vi "StateDrivebase.vi"(0 "Master State":T1(ring)) -> ()   [LabVIEW 2019]
doc: "This VI performs all of the calculations and decisions related to the swerve drive. Driver profiles are tuned from this front panel."
uses:
  <vilib>/Rock Robotics/WPI/DriverStation/WPI_DriverStationRobotMode2.ctl
  dscommands.vi
  constants.vi
  dsdata.vi
  sensors.vi
  outputs.vi
panel:
  in  "Manual Fudge Factor Auto Target (deg)":dbl=5.0
  in  "PID Tuning Heading Lock":T2={"Kp"=0.00045, "Ki"=0.0, "Kd"=0.0, "N-Diff"=3, "N-Int"=10, "Int Error Window"=90.0, "Max Ouput"=1.0, "Min Output"=-1.0, "Square Derivative"=FALSE, "N-Prop"=5} {"N-Prop" min=1; "Int Error Window" min=0.0; "N-Int" min=2; "N-Diff" min=2; "Kd" min=0.0; "Ki" min=0.0; "Kp" min=0.0}
  in  "Deceleration Hysteresis (ms)":u32=1
  out "Heading Control":bool
  in  "Heading Lock Strafe Deadband (ft/s)":dbl=3.0
  in  "Manually Disable Heading Lock":bool
  in  "PID Tuning Feeder Station":T3={"Kp"=0.0045, "Ki"=0.01, "Kd"=0.0002, "N-Diff"=10, "N-Int"=10, "Int Error Window"=30.0, "Max Ouput"=1.0, "Min Output"=-1.0} {"Int Error Window" min=0.0; "N-Int" min=2; "N-Diff" min=2; "Kd" min=0.0; "Ki" min=0.0; "Kp" min=0.0}
  out "Heading Controller Summary":T4(graph)
  in  "PID Tuning Auto Targeting":T3={"Kp"=0.006, "Ki"=0.0, "Kd"=0.0002, "N-Diff"=10, "N-Int"=10, "Int Error Window"=30.0, "Max Ouput"=0.4, "Min Output"=-0.4} {"Int Error Window" min=0.0; "N-Int" min=2; "N-Diff" min=2; "Kd" min=0.0; "Ki" min=0.0; "Kp" min=0.0}
  in  "Manual Fudge Factor Feeder Station(deg)":dbl=10.0
  in  "Plot Heading PID":bool
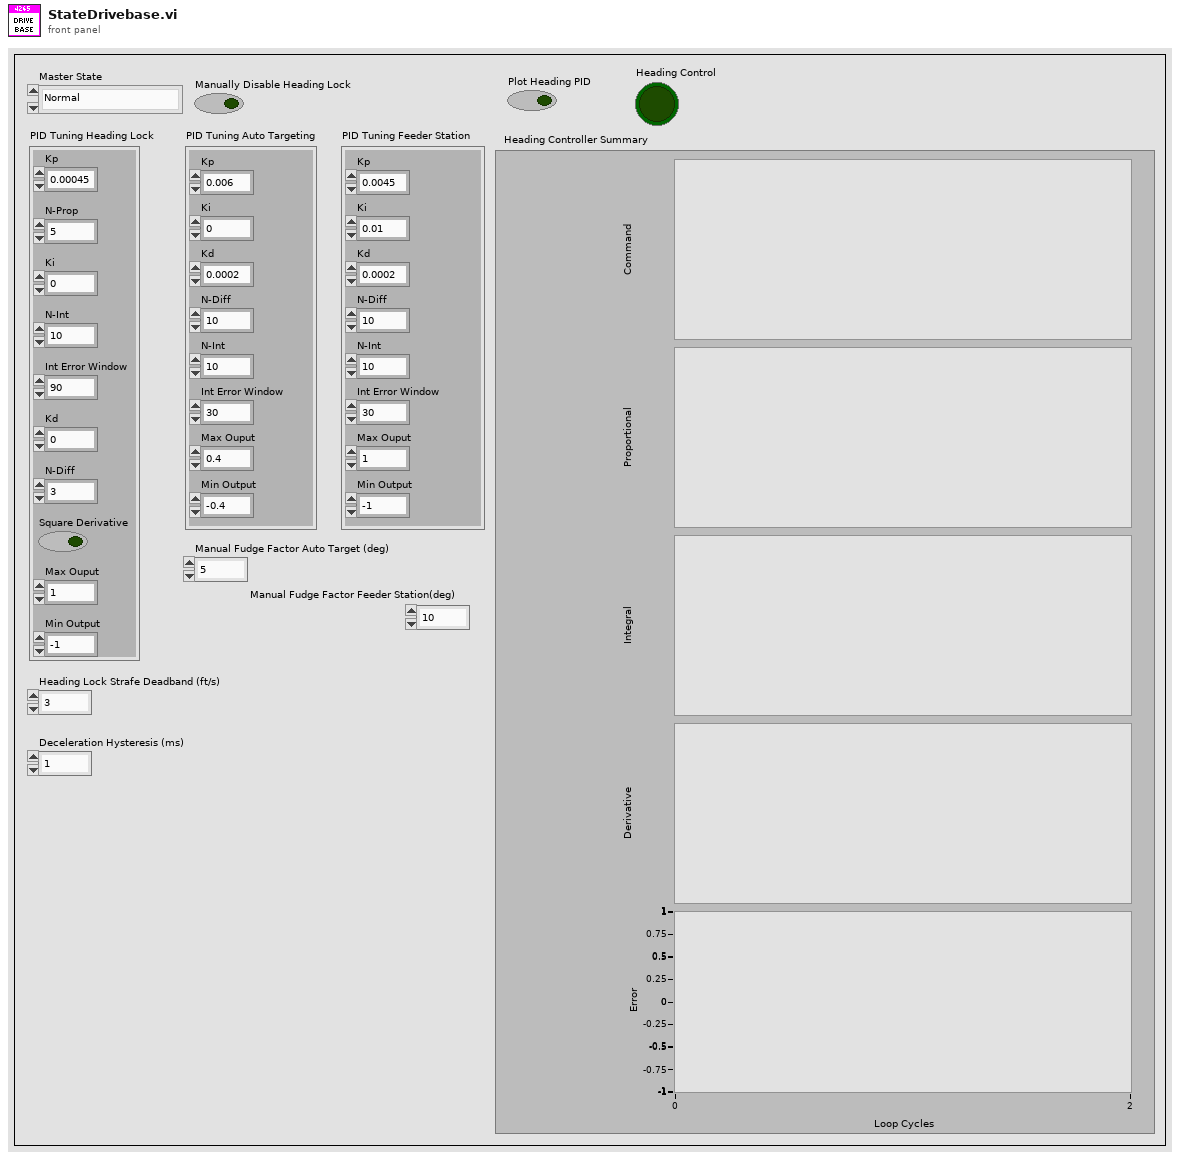
[diagram p1: front panel]
types:
  T1 = enum16{"Normal", "Control Rotation", "Control Position", "Climb"}
  T2 = cluster{"Kp":dbl, "Ki":dbl, "Kd":dbl, "N-Diff":i32, "N-Int":i32, "Int Error Window":dbl, "Max Ouput":dbl, "Min Output":dbl, "Square Derivative":bool, "N-Prop":i32}
  T3 = cluster{"Kp":dbl, "Ki":dbl, "Kd":dbl, "N-Diff":i32, "N-Int":i32, "Int Error Window":dbl, "Max Ouput":dbl, "Min Output":dbl}
  T4 = cluster{"Command":dbl, "Proportional":dbl, "Integral":dbl, "Derivative":dbl, "Goal":dbl}
  T5 = enum16{"Driver Control", "Auto Targeting", "Feeder Station"}
  T6 = typedef "WPI_DriverStationRobotMode2.ctl" = enum16{"Autonomous Disabled", "Autonomous Enabled", "Teleop Disabled", "Teleop Enabled", "Disconnected", "Finish", "Test Disabled", "Test Enabled", "Emergency Stopped"}
  T7 = cluster{"Current Setpoints[0]":dbl, "Current Setpoints[1]":dbl, "Current Setpoints[2]":dbl, "Current Setpoints[3]":dbl, "Current Setpoints[4]":dbl, "Current Setpoints[5]":dbl, "Current Setpoints[6]":dbl, "Current Setpoints[7]":dbl, "Current Setpoints[8]":dbl}
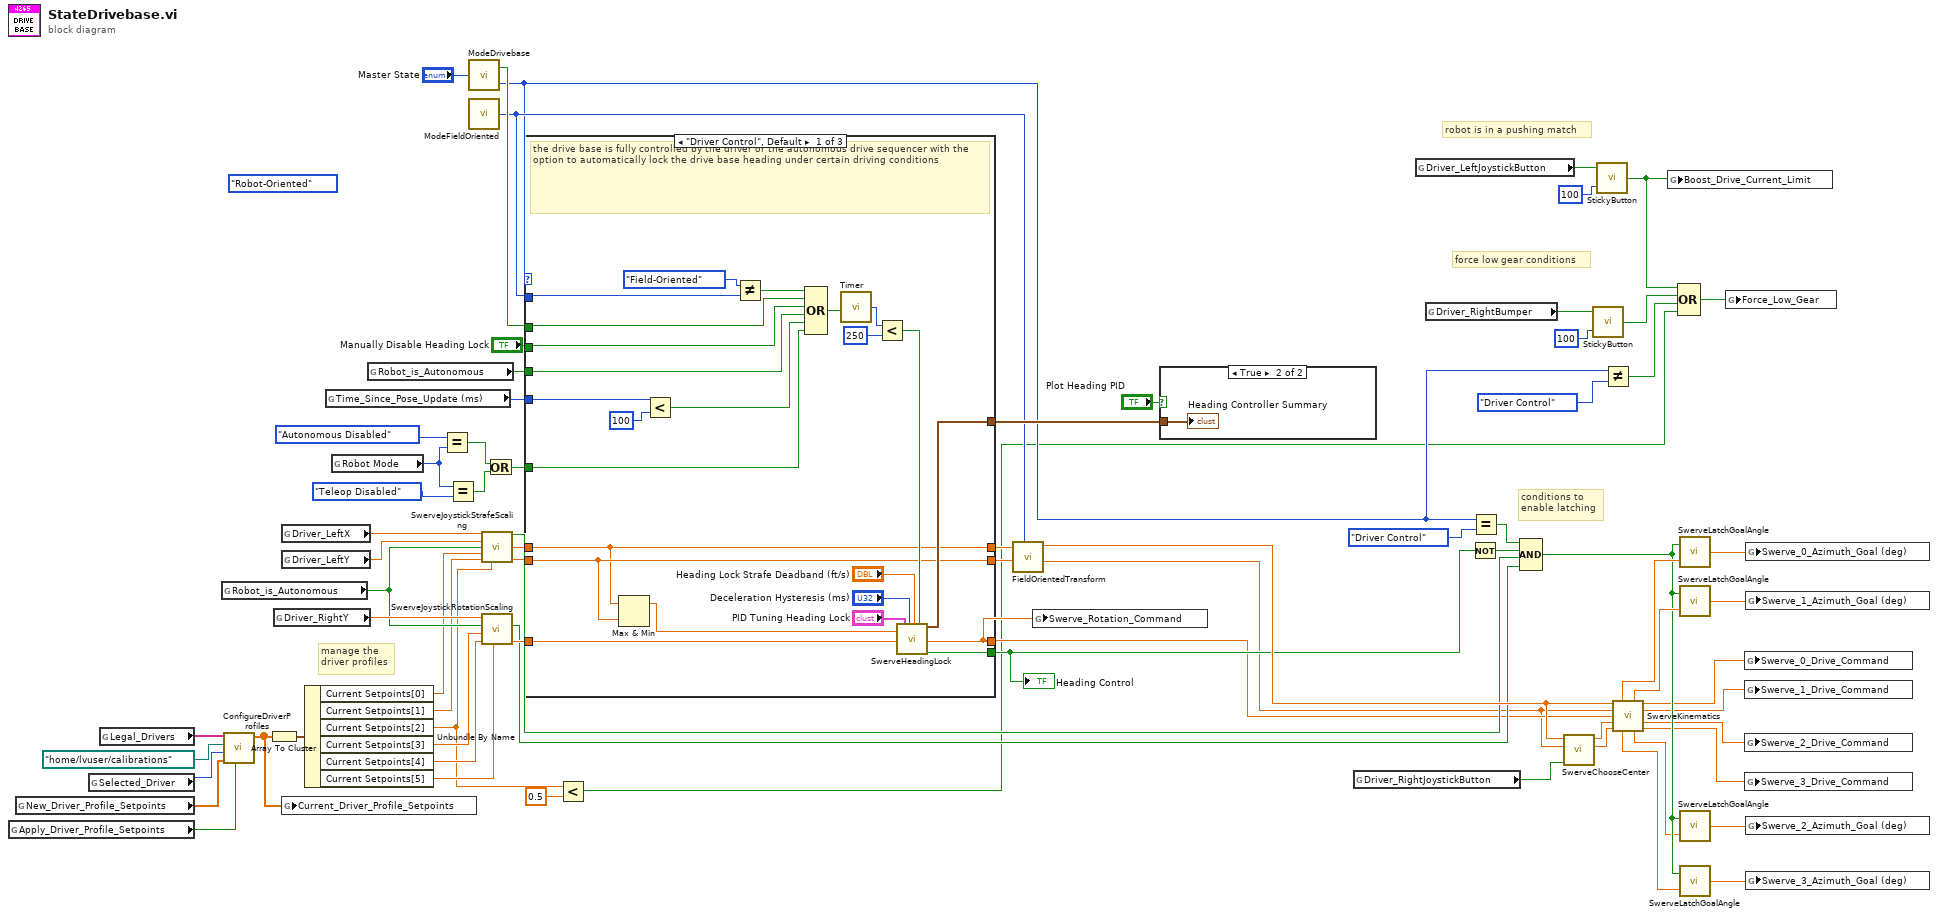
[diagram p0: block diagram]
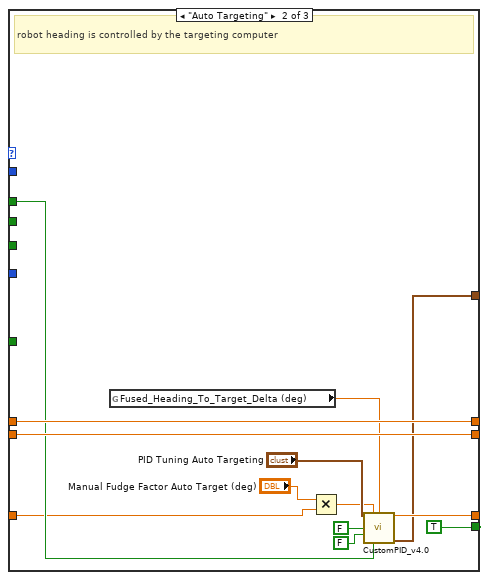
[diagram p3: hidden frame]
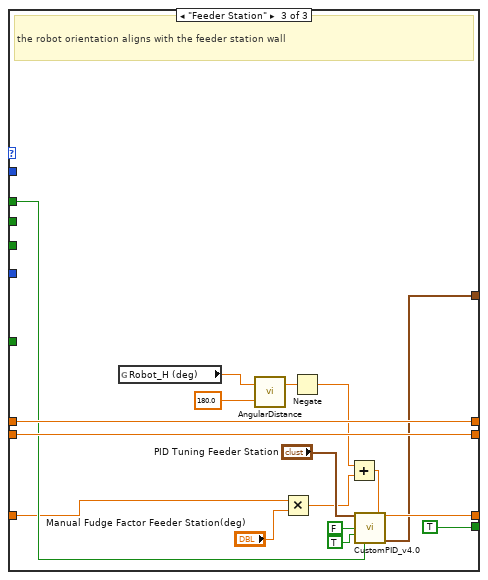
[diagram p4: hidden frame]
diagram:
  (unwired) enum16{"Robot-Oriented", "Field-Oriented"}."Robot-Oriented" ("Orientation Mode")
  # "force low gear conditions"
  # "robot is in a pushing match"
  # "conditions to\nenable latching"
  # "manage the\ndriver profiles"
  n1 = global read "dsdata.vi" "Apply_Driver_Profile_Setpoints"() -> (w7:bool)
  n2 = global read "dsdata.vi" "New_Driver_Profile_Setpoints"() -> (w9:dbl[])
  n3 = global read "dsdata.vi" "Selected_Driver"() -> (w8:i32)
  n4 = global read "constants.vi" "Legal_Drivers"() -> (w11:string[])
  n5 = global read "dsdata.vi" "Robot_is_Autonomous"() -> (w52:bool)
  n6 = call "ConfigureDriverProfiles.vi"("Apply New Setpoint"=w7, "New Setpoints"=w9, "Selected Driver"=w8, "Setpoint Save Location"=path "/home/lvuser/calibrations", "Driver Profile Names"=w11) -> ("Current Setpoints"=w6:dbl[])  [unwired: 6 in]
  n7 = Array To Cluster(array=w6) -> (cluster=w5:T7)
  n8 = global read "dscommands.vi" "Driver_RightY"() -> (w53:dbl)
  n9 = global read "dscommands.vi" "Driver_LeftX"() -> (w58:dbl)
  n10 = global read "dscommands.vi" "Driver_LeftY"() -> (w57:dbl)
  n11 = global write "outputs.vi" "Current_Driver_Profile_Setpoints"(w6) -> ()
  n12 = Unbundle By Name(w5) -> ("Current Setpoints[0]"=w40:dbl, "Current Setpoints[1]"=w39:dbl, "Current Setpoints[2]"=w3:dbl, "Current Setpoints[3]"=w24:dbl, "Current Setpoints[4]"=w23:dbl, "Current Setpoints[5]"=w22:dbl)
  n13 = global read "sensors.vi" "Time_Since_Pose_Update (ms)"() -> (w66:u32)
  n14 = global read "dsdata.vi" "Robot Mode"() -> (w29:T6)
  n15 = global read "dsdata.vi" "Robot_is_Autonomous"() -> (w65:bool)
  n16 = Equal?(x=WPI_DriverStationRobotMode2."Autonomous Disabled" ("Robot Mode"), y=w29) -> (x = y?=w27:bool)
  n17 = Equal?(x=w29, y=WPI_DriverStationRobotMode2."Teleop Disabled" ("Robot Mode")) -> (x = y?=w26:bool)
  n18 = call "ModeDrivebase.vi"("Master State"="Master State") -> ("Drive Mode Change"=w63:bool, "Drive Mode"=w14:T5)
  n19 = call "ModeFieldOriented.vi"() -> ("Orientation Mode"=w42:enum16{"Robot-Oriented", "Field-Oriented"})  [unwired: 1 in]
  n20 = call "SwerveJoystickStrafeScaling.vi"("Raw Joystick X"=w58, "Raw Joystick Y"=w57, "Auto Control"=w52, "Strafe Deadband"=w40, "Strafe Scaling"=w39, "Strafe Maximum"=w3) -> ("In Deadband"=w48:bool, "Scaled Joystick X"=w56:dbl, "Scaled Joystick Y"=w55:dbl)  [unwired: 7 in]
  n21 = call "SwerveJoystickRotationScaling.vi"("Rotation Maximum"=w22, "Rotation Scaling"=w23, "Rotation Deadband"=w24, "Auto Control"=w52, "Raw Joystick Rotation"=w53) -> ("Scaled Joystick Rotation"=w54:dbl, "In Deadband"=w49:bool)  [unwired: 4 in]
  n22 = Or(x=w27, y=w26) -> (x .or. y?=w25:bool)
  n23 = case shown="\"Driver Control\", Default" w14 {
    tunnel: [w76 w109 w125] -> w41
    tunnel: [w75 w110 w123] -> w73
    tunnel: w56 -> [w75 w110 w123]
    tunnel: w55 -> [w76 w109 w125]
    tunnel: w54 -> [w87 w99 w115]
    tunnel: [w88 w101 w122] -> w47
    tunnel: [w93 TRUE ("auto rot control") TRUE ("auto rot control")] -> w50
    tunnel: w42 -> [w94 _ _]
    tunnel: w65 -> [w91 _ _]
    tunnel: w63 -> [w85 w104 w118]
    tunnel: w66 -> [w97 _ _]
    tunnel: [w90 w100 w117] -> w64
    tunnel: "Manually Disable Heading Lock" -> [w89 _ _]
    tunnel: w25 -> [w79 _ _]
    frame "Driver Control", Default {
      # "the drive base is fully controlled by the driver or the autonomous drive sequencer with the option to automatically lock the drive base heading under certain driving conditions"
      n24 = Max & Min(x=w75, y=w76) -> (max(x,y)=w74:dbl)  [unwired: 1 out]
      n25 = Less?(x=w97, y=u32 100) -> (x < y?=w92:bool)
      n26 = Not Equal?(x=enum16{"Robot-Oriented", "Field-Oriented"}."Field-Oriented" ("Orientation Mode"), y=w94) -> (x != y?=w84:bool)
      n27 = Compound Arithmetic op=OR(w84, w85, w89, w91, w92, w79) -> (w82:bool)
      n28 = call "Timer.vi"("Reset Timer"=w82) -> ("Time (ms)"=w83:u32)
      n29 = Less?(x=w83, y=u32 250) -> (x < y?=w80:bool)
      n30 = call "SwerveHeadingLock.vi"("Max Driver Translation Joystick"=w74, "Driver Rotation Joystick"=w87, "PID Tuning Parameters"="PID Tuning Heading Lock", "Deceleration Hysteresis (ms)"="Deceleration Hysteresis (ms)", "Heading Lock Strafe Deadband (ft/s)"="Heading Lock Strafe Deadband (ft/s)", "External Disables"=w80) -> ("Controller Summary"=w90:T4, "Joystick Rotation"=w88:dbl, "Heading Lock"=w93:bool)  [unwired: 11 in]
    }
    frame "Auto Targeting" {
      # "robot heading is controlled by the targeting computer"
      n31 = global read "sensors.vi" "Fused_Heading_To_Target_Delta (deg)"() -> (w105:dbl)
      n32 = Multiply(x="Manual Fudge Factor Auto Target (deg)", y=w99) -> (x*y=w106:dbl)
      n33 = call "CustomPID_v4.0.vi"("PID Tuning Parameters"="PID Tuning Auto Targeting", "Goal"=w106, "Process Variable"=w105, "Reset on Goal Change ?"=FALSE, "Use Custom Error Calculation ?"=FALSE, "Reinit"=w104) -> ("Command"=w101:dbl, "Controller Summary"=w100:T4)  [unwired: 6 in, 2 out]
    }
    frame "Feeder Station" {
      # "the robot orientation aligns with the feeder station wall"
      n34 = global read "sensors.vi" "Robot_H (deg)"() -> (w127:dbl)
      n35 = call "AngularDistance.vi"("Goal Angle (deg) [0,360]"=180.0, "Current Angle (deg) [-Inf,+Inf]"=w127) -> ("Signed Angular Distance (deg) [-180,+180]"=w116:dbl)  [unwired: 1 out]
      n36 = Multiply(x=w115, y="Manual Fudge Factor Feeder Station(deg)") -> (x*y=w114:dbl)
      n37 = Negate(x=w116) -> (-x=w113:dbl)
      n38 = Add(x=w113, y=w114) -> (x+y=w112:dbl)
      n39 = call "CustomPID_v4.0.vi"("PID Tuning Parameters"="PID Tuning Feeder Station", "Custom Error Calculation"=w112, "Reset on Goal Change ?"=FALSE, "Use Custom Error Calculation ?"=TRUE, "Reinit"=w118) -> ("Command"=w122:dbl, "Controller Summary"=w117:T4)  [unwired: 7 in, 2 out]
    }
  }
  "Heading Control" <- w50
  n40 = Less?(x=w3, y=0.5) -> (x < y?=w1:bool)
  n41 = call "FieldOrientedTransform.vi"("Orientation Mode"=w42, "Joystick Y"=w41, "Joystick X"=w73) -> ("Joystick Y'"=w43:dbl, "Joystick X'"=w51:dbl)  [unwired: 7 in]
  n42 = global write "outputs.vi" "Swerve_Rotation_Command"(w47) -> ()
  n43 = case shown="True" "Plot Heading PID" {
    tunnel: w64 -> [_ w128]
    frame False {
    }
    frame True {
      "Heading Controller Summary" <- w128
    }
  }
  n44 = global read "dscommands.vi" "Driver_RightJoystickButton"() -> (w62:bool)
  n45 = global read "dscommands.vi" "Driver_LeftJoystickButton"() -> (w60:bool)
  n46 = global read "dscommands.vi" "Driver_RightBumper"() -> (w21:bool)
  n47 = Not(x=w50) -> (.not. x?=w46:bool)
  n48 = Equal?(x=w14, y=T5."Driver Control" ("x")) -> (x = y?=w45:bool)
  n49 = Compound Arithmetic op=AND(w45, w46, w48, w49) -> (w69:bool)
  n50 = call "SwerveChooseCenter.vi"("Defensive Driving Trigger"=w62, "Joystick Y"=w43, "Joystick X"=w51) -> ("Cy (in)"=w12:dbl, "Cx (in)"=w13:dbl)  [unwired: 5 in]
  n51 = call "StickyButton.vi"("Time threshold (ms)"=u32 100 ("y"), "Button Input"=w21) -> ("Sticky Button"=w18:bool)
  n52 = call "StickyButton.vi"("Time threshold (ms)"=u32 100 ("y"), "Button Input"=w60) -> ("Sticky Button"=w19:bool)
  n53 = Not Equal?(x=w14, y=T5."Driver Control") -> (x != y?=w15:bool)
  n54 = call "SwerveKinematics.vi"("Joystick X"=w51, "Joystick Y"=w43, "Joystick Rotation"=w47, "Cx (in)"=w13, "Cy (in)"=w12) -> ("Module 0 Angle (deg)"=w72:dbl, "Module 1 Angle (deg)"=w71:dbl, "Module 0 Velocity Command (ul)"=w38:dbl, "Module 1 Velocity Command (ul)"=w37:dbl, "Module 2 Velocity Command (ul)"=w36:dbl, "Module 3 Angle (deg)"=w67:dbl, "Module 2 Angle (deg)"=w68:dbl, "Module 3 Velocity Command (ul)"=w35:dbl)  [unwired: 3 in]
  n55 = global write "outputs.vi" "Boost_Drive_Current_Limit"(w19) -> ()
  n56 = Compound Arithmetic op=OR(w19, w18, w15, w1) -> (w17:bool)
  n57 = call "SwerveLatchGoalAngle.vi"("Raw Goal Angle"=w72, "In Deadband"=w69) -> ("Latched Goal Angle"=w34:dbl)
  n58 = call "SwerveLatchGoalAngle.vi"("Raw Goal Angle"=w71, "In Deadband"=w69) -> ("Latched Goal Angle"=w33:dbl)
  n59 = call "SwerveLatchGoalAngle.vi"("Raw Goal Angle"=w68, "In Deadband"=w69) -> ("Latched Goal Angle"=w32:dbl)
  n60 = call "SwerveLatchGoalAngle.vi"("Raw Goal Angle"=w67, "In Deadband"=w69) -> ("Latched Goal Angle"=w31:dbl)
  n61 = global write "outputs.vi" "Force_Low_Gear"(w17) -> ()
  n62 = global write "outputs.vi" "Swerve_0_Drive_Command"(w38) -> ()
  n63 = global write "outputs.vi" "Swerve_1_Drive_Command"(w37) -> ()
  n64 = global write "outputs.vi" "Swerve_2_Drive_Command"(w36) -> ()
  n65 = global write "outputs.vi" "Swerve_3_Drive_Command"(w35) -> ()
  n66 = global write "outputs.vi" "Swerve_0_Azimuth_Goal (deg)"(w34) -> ()
  n67 = global write "outputs.vi" "Swerve_1_Azimuth_Goal (deg)"(w33) -> ()
  n68 = global write "outputs.vi" "Swerve_2_Azimuth_Goal (deg)"(w32) -> ()
  n69 = global write "outputs.vi" "Swerve_3_Azimuth_Goal (deg)"(w31) -> ()
